vi "SendString.vi"(8 "error in (no error)":errorcluster, 10 "String":string, 11 "StringReader in":refnum<class "StringReader.lvclass">) -> (0 "error out":errorcluster, 3 "StringReader out":refnum<class "StringReader.lvclass">)   [LabVIEW 2013, in "StringReader.lvclass"]
doc: "Send a string to the remote destination"
uses:
  StringReader.lvclass
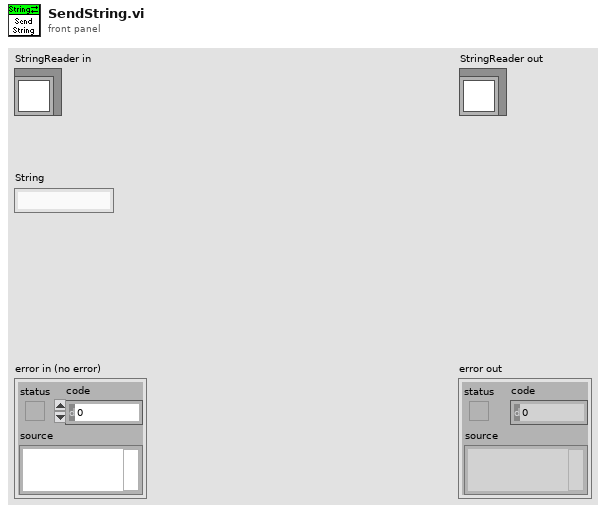
[diagram p1: front panel]
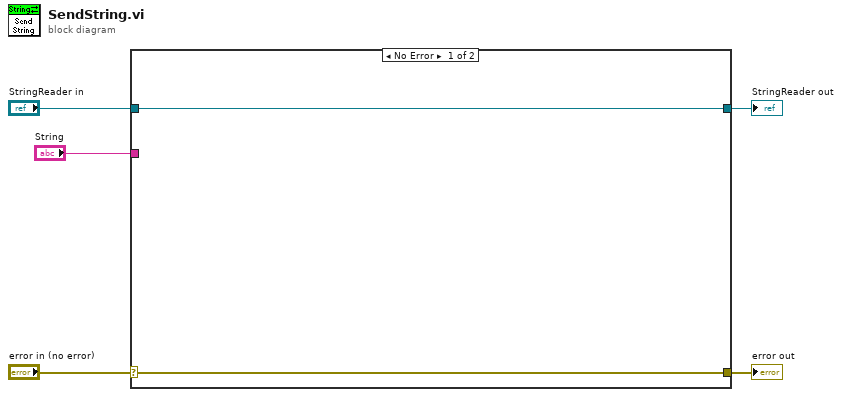
[diagram p0: block diagram]
diagram:
  n1 = case shown="No Error" "error in (no error)" {
    selector: "error in (no error)" -> [w6 w9]
    tunnel: [w6 w9] -> w4
    tunnel: [w7 w8] -> w2
    tunnel: "StringReader in" -> [w7 w8]
    tunnel: "String" -> [_ _]
    frame No Error {
    }
    frame Error {
    }
  }
  "error out" <- w4
  "StringReader out" <- w2
